vi "niScope EX Configured Acquisition_V3.vi"() -> ()   [LabVIEW 2024]
doc: "Recommended Input Signal: 100 kHz, 4 Vpp, sine wave\n\nDevices Supported: Refer to NI Example Finder\n\nThis example configures all the oscilloscope's vertical, horizontal, and triggering properties before every acquisition. It allows you to experiment with numerous configurations, including acquisition types and triggering modes, since it supports nearly the entire functionality of NI-SCOPE. However, it is may be more instructive to consult other examples about specific topics such as FlexRes, Random Interleaved Sampling, and Multi-Record to learn more about these features.\n\nMany parameters are included an the front panel of this example. Notice that the \"min sample rate\" is next to the \"actual sample rate,\" and similarly the \"min record length\" is near the \"actual record length.\" The \"min\" values are specified with the Configure Horizontal Timing VI. NI-SCOPE maintains a constant time per record for each acquisition. So when you specify a min sample rate and a min record length, this determines the amount of time the acquisition should take:\n\n time per record = min record length / min sampling rate. \n\nHowever, oscilloscopes support only a certain number of defined sampling rates, so if the value chosen is not a valid rate, it is rounded to the next higher rate, called the actual sample rate. The actual record length is then calculated in order to maintain the time per record. Both of these values are returned in this example so you can investigate the effects of parameter rounding with your oscilloscope. For more information about parameter coercions, see the NI High Speed Digitizers Help.\n\nThe enforce realtime property allows this example to use Random Interleaved Sampling. See the Random Interleaved Sampling example for more details.\n\nKeep in mind that not all digitizers/oscilloscopes support all the features in this example. The NI High Speed Digitizers Help includes a table of supported features for each device."
uses:
  <instrlib>/niScope/Controls/niScope vertical coupling.ctl
  <instrlib>/niScope/Utility/niScope Get Channel Name From String.vi
  <instrlib>/niScope/Configure/Trigger/niScope Configure Trigger Immediate.vi
  <instrlib>/niScope/Configure/Trigger/niScope Configure Trigger Edge.vi
  <instrlib>/niScope/Configure/Trigger/niScope Configure Trigger Digital.vi
  <instrlib>/niScope/Configure/Trigger/niScope Configure Trigger Window.vi
  <instrlib>/niScope/Configure/Trigger/niScope Configure Trigger Hysteresis.vi
  <instrlib>/niScope/Acquire/Fetch/niScope Multi Fetch WDT.vi
panel:
  out "Waveform Graph 2":waveform(dbl)(graph)
  out "Waveform Graph":waveform(dbl)(graph)
  in  "Trigger Type":T1(tab)
  in  "Trigger Source":string(combo)="0"
  in  "Trigger Level":dbl format="%.2f"
  in  "Trigger Slope":i32(ring) items=["Positive", "Negative"]
  in  "Coupling":u16(ring)=1 caption="Trigger Coupling" items=["AC"=0, "DC"=1, "HF Reject"=3, "LF Reject"=4, "AC Plus HF Reject"=1001]
  in  "Trigger Slope":i32(ring) items=["Positive", "Negative"]
  in  "Trigger Source":string(combo)="VAL_PFI_1"
  in  "Coupling":u16(ring)=1 caption="Trigger Coupling" items=["AC"=0, "DC"=1, "HF Reject"=3, "LF Reject"=4, "AC Plus HF Reject"=1001]
  in  "High Level":dbl=0.1 caption="Window High Level" format="%.2f"
  in  "Low Level":dbl=-0.1 caption="Window Low Level" format="%.2f"
  in  "Window Mode":i32(ring) items=["Entering", "Leaving"]
  in  "Trigger Source":string(combo)="0"
  in  "Hysteresis":dbl=0.05 format="%.2f"
  in  "Trigger Source":string(combo)="0"
  in  "Trigger Level":dbl format="%.2f"
  in  "Coupling":u16(ring)=1 caption="Trigger Coupling" items=["AC"=0, "DC"=1, "HF Reject"=3, "LF Reject"=4, "AC Plus HF Reject"=1001]
  in  "Trigger Slope":i32(ring) items=["Positive", "Negative"]
  out "Auto Triggered":bool
  in  "Trigger Modifier":i32(ring)=2 items=["None"=1, "Auto Trigger"=2]
  in  "Stop":bool
  in  "Reference Position":dbl=50.0 caption="Ref Position" format="%.1f"
  in  "Trigger Delay":dbl caption="Trigger Delay (s)" format="%#.4p"
  in  "Maximum Input Frequency":dbl caption="Max. Input Frequency (Hz)" format="%.2f"
  in  "Input Impedance":u32(ring) items=["1 mega ohm"=0, "50 ohms"=2]
  in  "Vertical Offset":dbl caption="Vertical Offset (V)" format="%.2p"
  out "Actual Sample Rate":dbl=10000000.0 format="%#.2p"
  out "Actual Record Length":i32=1000
  in  "Min Record Length":i32=1000 caption="Min. Record Length"
  in  "Min Sample Rate":dbl=10000000.0 caption="Min. Sample Rate" step=1000000.0 format="%#.2p"
  in  "Vertical Range":dbl=5.0 caption="Vertical Range (V)" format="%.2f"
  in  "Enforce Realtime":bool=TRUE
  in  "Channel Name":string="0" caption="Channel(s)"
  in  "Resource Name":refnum<k15>="Dev1" caption="Resource Name(s)"
  # "Vertical"
  # "Channel"
  # "Trigger"
  # "Common Trigger Settings"
  # "Horizontal"
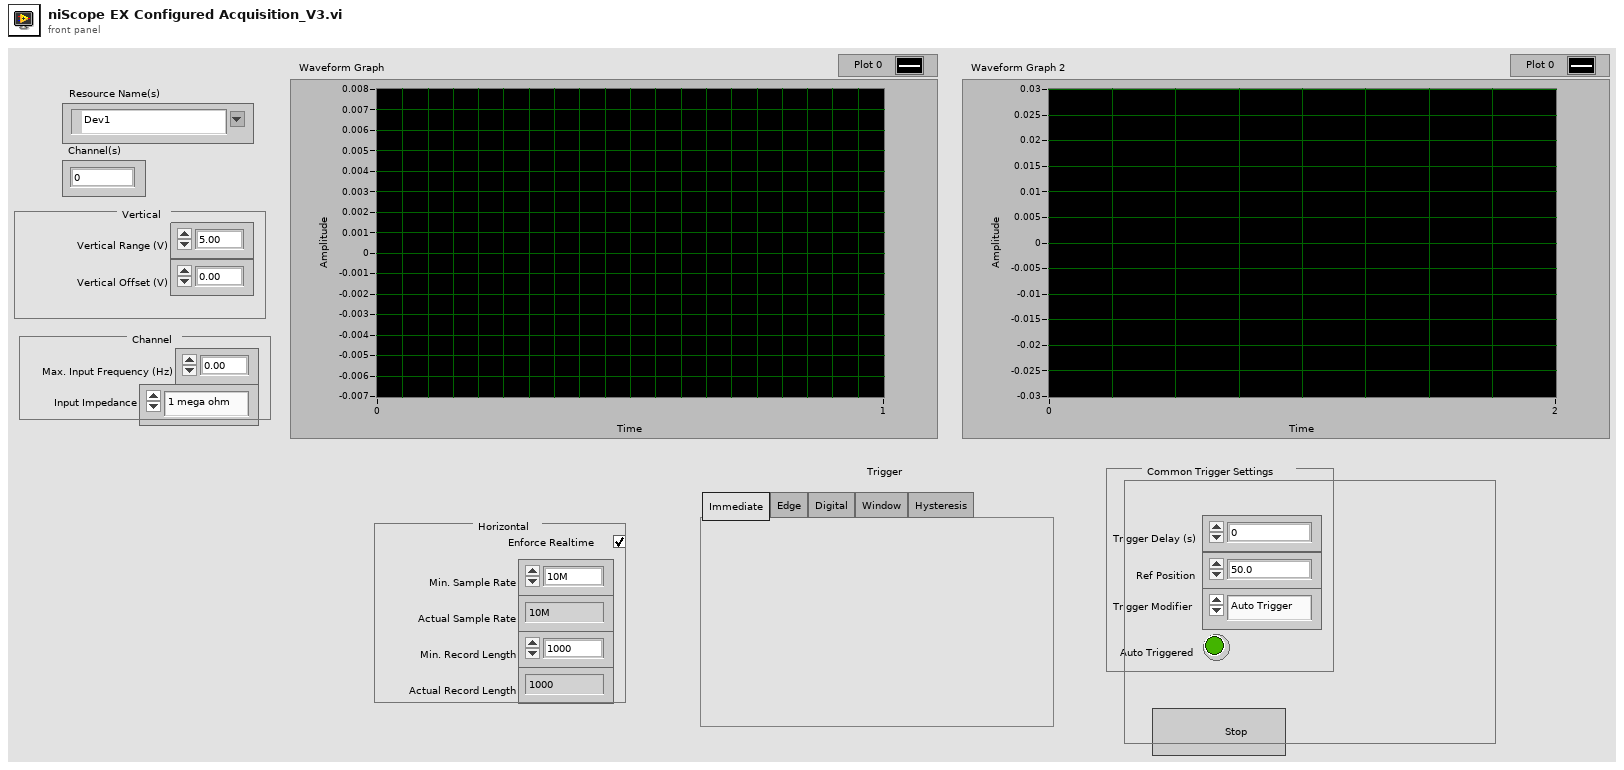
[diagram p1: front panel]
types:
  T1 = enum32{"Immediate", "Edge", "Digital", "Window", "Hysteresis"}
  T2 = enum16{"open", "open or create", "create or replace", "create", "open (read-only)"}
  T3 = typedef "niScope vertical coupling.ctl" = i32
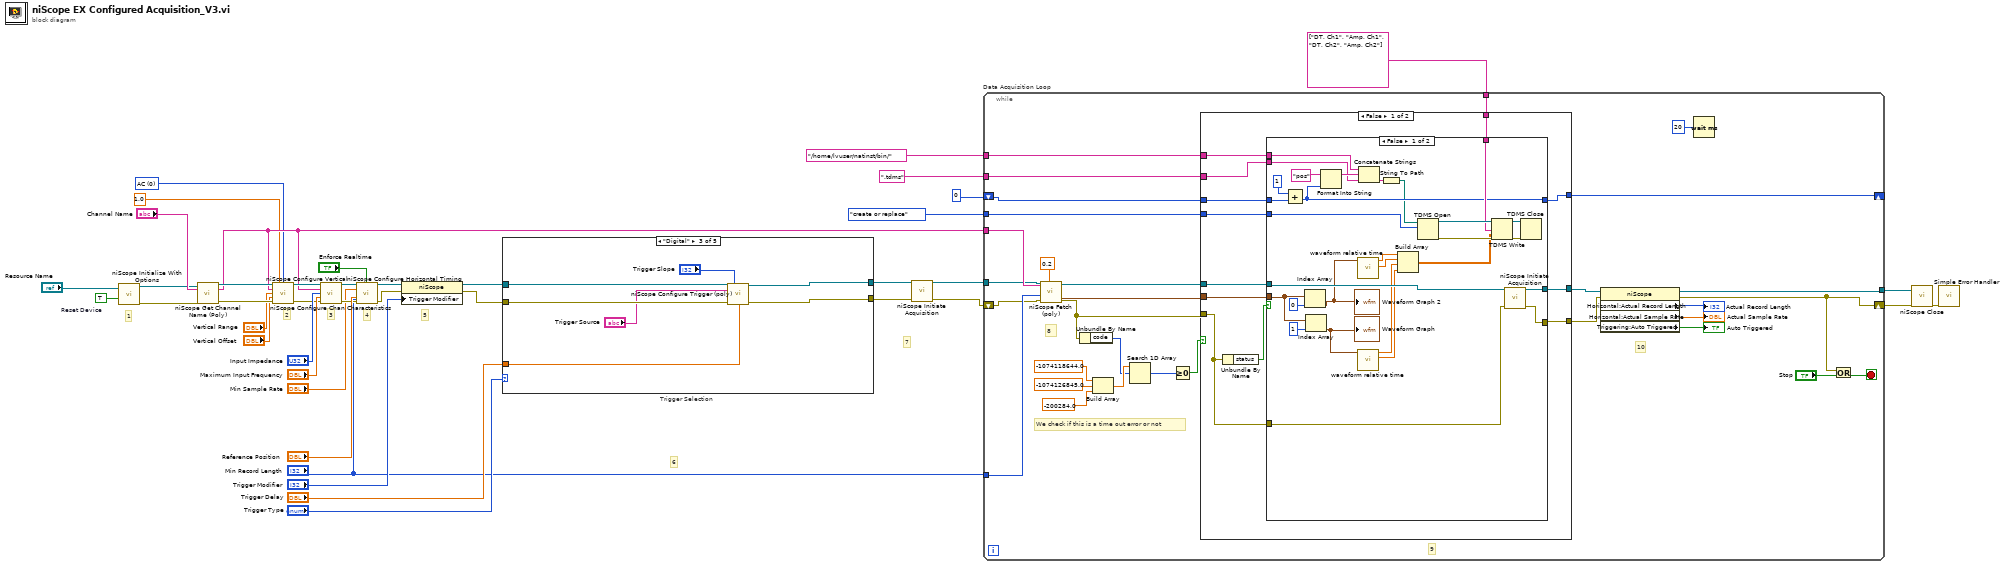
[diagram p0: block diagram]
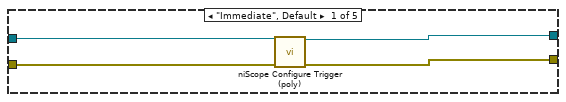
[diagram p2: hidden frame]
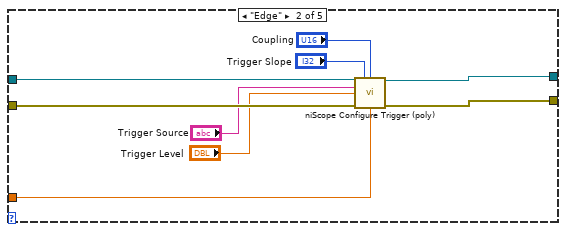
[diagram p3: hidden frame]
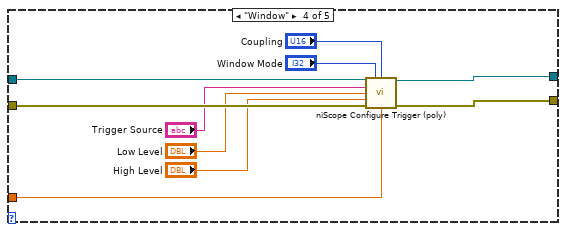
[diagram p4: hidden frame]
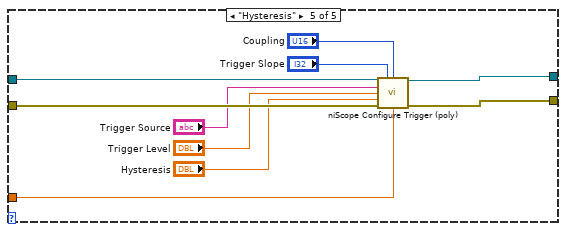
[diagram p5: hidden frame]
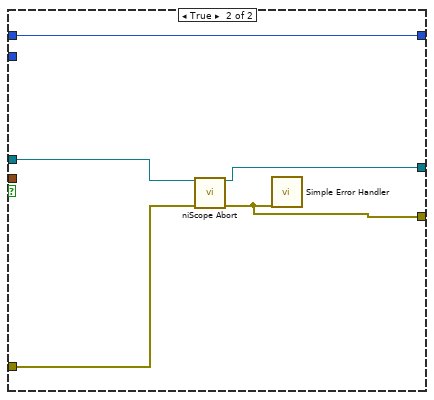
[diagram p6: hidden frame]
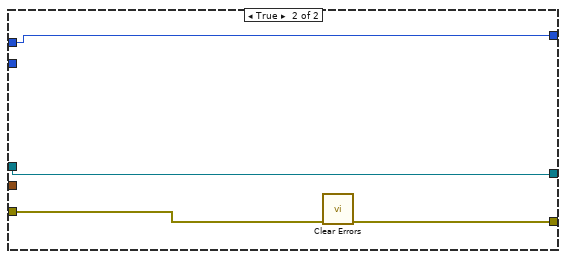
[diagram p7: hidden frame]
diagram:
  w7 = T3 0 items=["AC", "DC", "Ground"] ("vertical coupling")
  w41 = TRUE  # Reset Device
  # "5"
  # "2"
  # "3"
  # "4"
  # "6"
  # "7"
  # "1"
  n1 = call <instrlib>:"niScope Initialize With Options.vi"("resource name"="Resource Name", "reset device"=w41) -> ("instrument handle"=w13:refnum<k15>, "error out"=w12:errorcluster)  [unwired: 12 in]
  n2 = call-poly <instrlib>:"niScope Get Channel Name (Poly).vi"("instrument handle"=w13, "index"="Channel Name", "error in"=w12) -> ("instrument handle out"=w34:refnum<k15>, "channel name"=w11:string, "error out"=w35:errorcluster)  [unwired: 10 in]
  n3 = call <instrlib>:"niScope Configure Vertical.vi"("instrument handle"=w34, "probe attenuation"=1.0, "vertical coupling"=w7, "channels"=w11, "vertical range"="Vertical Range", "vertical offset"="Vertical Offset", "error in"=w35) -> ("instrument handle out"=w16:refnum<k15>, "error out"=w17:errorcluster)  [unwired: 7 in]
  n4 = call <instrlib>:"niScope Configure Chan Characteristics.vi"("instrument handle"=w16, "channels"=w11, "input impedance"="Input Impedance", "maximum input frequency"="Maximum Input Frequency", "error in"=w17) -> ("instrument handle out"=w19:refnum<k15>, "error out"=w18:errorcluster)  [unwired: 9 in]
  n5 = call <instrlib>:"niScope Configure Horizontal Timing.vi"("instrument handle"=w19, "enforce realtime"="Enforce Realtime", "min sample rate"="Min Sample Rate", "reference position"="Reference Position", "error in"=w18, "min record length"="Min Record Length") -> ("instrument handle out"=w27:refnum<k15>, "error out"=w28:errorcluster)  [unwired: 8 in]
  n6 = property on="Property Node" class="niScope"(reference=w27, error in=w28, "Trigger Modifier"="Trigger Modifier") -> (reference out=w30:refnum<k15>, error out=w29:errorcluster)
  n7 = case "Trigger Selection" shown="\"Digital\"" "Trigger Type" {
    tunnel: w29 -> [w45 w54 w61 w71 w81]
    tunnel: [w42 w50 w57 w67 w77] -> w26
    tunnel: w30 -> [w44 w53 w60 w70 w80]
    tunnel: [w43 w51 w58 w68 w79] -> w25
    tunnel: "Trigger Delay" -> [_ w52 w59 w69 w78]
    frame "Immediate", Default {
      n8 = call-poly <instrlib>:"niScope Configure Trigger (poly).vi"("instrument handle"=w44, "error in"=w45) -> ("instrument handle out"=w43:refnum<k15>, "error out"=w42:errorcluster)  [unwired: 12 in]
    }
    frame "Edge" {
      n9 = call-poly <instrlib>:"niScope Configure Trigger (poly).vi"("instrument handle"=w53, "trigger slope"="Trigger Slope", "trigger coupling"="Coupling", "trigger source"="Trigger Source", "trigger level"="Trigger Level", "error in"=w54, "trigger delay"=w52) -> ("instrument handle out"=w51:refnum<k15>, "error out"=w50:errorcluster)  [unwired: 7 in]
    }
    frame "Digital" {
      n10 = call-poly <instrlib>:"niScope Configure Trigger (poly).vi"("instrument handle"=w60, "trigger slope"="Trigger Slope", "trigger source"="Trigger Source", "error in"=w61, "trigger delay"=w59) -> ("instrument handle out"=w58:refnum<k15>, "error out"=w57:errorcluster)  [unwired: 9 in]
    }
    frame "Window" {
      n11 = call-poly <instrlib>:"niScope Configure Trigger (poly).vi"("instrument handle"=w70, "trigger window mode"="Window Mode", "trigger coupling"="Coupling", "trigger source"="Trigger Source", "low level"="Low Level", "high level"="High Level", "error in"=w71, "trigger delay"=w69) -> ("instrument handle out"=w68:refnum<k15>, "error out"=w67:errorcluster)  [unwired: 6 in]
    }
    frame "Hysteresis" {
      n12 = call-poly <instrlib>:"niScope Configure Trigger (poly).vi"("instrument handle"=w80, "trigger slope"="Trigger Slope", "trigger coupling"="Coupling", "trigger source"="Trigger Source", "trigger level"="Trigger Level", "hysteresis"="Hysteresis", "error in"=w81, "trigger delay"=w78) -> ("instrument handle out"=w79:refnum<k15>, "error out"=w77:errorcluster)  [unwired: 6 in]
    }
  }
  n13 = call <instrlib>:"niScope Initiate Acquisition.vi"("instrument handle"=w25, "error in"=w26) -> ("instrument handle out"=w10:refnum<k15>, "error out"=w8:errorcluster)  [unwired: 12 in]
  n14 = while "Data Acquisition Loop" {
    tunnel: [w112] -> w39
    shift-right: [w106] -> w38
    shift-left: w8 -> [w88]
    tunnel: w11 -> [w91]
    tunnel: w10 -> [w90]
    tunnel: "Min Record Length" -> [w89]
    tunnel: string[] ["DT, Ch1", "Amp, Ch1", "DT, Ch2", "Amp, Ch2"] ("channel name(s) in (Untitled)") -> [w87]
    tunnel: "/home/lvuser/natinst/bin/" ("string") -> [w86]
    tunnel: ".tdms" ("string") -> [w85]
    tunnel: T2."create or replace" ("operation (0:open)") -> [w84]
    shift-right: [w82] -> _
    shift-left: 0 -> [w83]
    stop <- w107 stop-if-true
    # "9"
    # "We check if this is a time out error or not"
    # "8"
    # "10"
    n15 = call-poly <instrlib>:"niScope Fetch (poly).vi"("timeout"=0.2, "error in"=w88, "numSamples"=w89, "channels"=w91, "instrument handle"=w90) -> ("error out"=w98:errorcluster, "wfm"=w94:waveform(dbl)[], "instrument handle out"=w96:refnum<k15>)  [unwired: 3 in, 1 out]
    n16 = Unbundle By Name(w98) -> ("code"=w92:i32)
    n17 = Build Array(-1074118644.0 ("element"), -1074126845.0 ("element"), -200284.0 ("element")) -> (w101:dbl[])
    n18 = Search 1D Array(1D array=w101, element=w92) -> (index of element=w100:i32)  [unwired: 1 in]
    n19 = Greater Or Equal To 0?(x=w100) -> (x >= 0?=w99:bool)
    n20 = case shown="False" w99 {
      tunnel: w98 -> [w120 w162]
      tunnel: [w123 w161] -> w97
      tunnel: w96 -> [w122 w161]
      tunnel: [w121 w160] -> w95
      tunnel: w94 -> [w119 _]
      tunnel: w87 -> [w118 _]
      tunnel: w86 -> [w115 _]
      tunnel: w85 -> [w114 _]
      tunnel: [w117 w159] -> w82
      tunnel: w84 -> [w116 _]
      tunnel: w83 -> [w113 w159]
      frame False {
        n21 = Unbundle By Name(w120) -> ("status"=w124:bool)
        n22 = case shown="False" w124 {
          tunnel: [w152 w157] -> w123
          tunnel: w122 -> [w153 w158]
          tunnel: [w150 w155] -> w121
          tunnel: w120 -> [w151 w156]
          tunnel: w119 -> [w141 _]
          tunnel: w118 -> [w148 _]
          tunnel: [w131 w154] -> w117
          tunnel: w116 -> [w129 _]
          tunnel: w115 -> [w128 _]
          tunnel: w114 -> [w127 _]
          tunnel: w113 -> [w126 w154]
          frame False {
            n23 = Add(x=1, y=w126) -> (x+y=w131:i32)
            n24 = Index Array(array=w141, index=0) -> (element=w136:waveform(dbl))
            "Waveform Graph 2" <- w136
            n25 = Index Array(array=w141, index=1) -> (element=w139:waveform(dbl))
            "Waveform Graph" <- w139
            n26 = Format Into String(initial string="pos", w131) -> (resulting string=w134:string)  [unwired: 2 in, 1 out]
            n27 = call "waveform relative time.vi"("signal in"=w136) -> ("Y"=w135:dbl[], "Relative Time"=w146:dbl[])  [unwired: 7 in, 2 out]
            n28 = call "waveform relative time.vi"("signal in"=w139) -> ("Y"=w137:dbl[], "Relative Time"=w138:dbl[])  [unwired: 7 in, 2 out]
            n29 = Concatenate Strings(w128, w134, w127) -> (w133:string)
            n30 = String To Path(string=w133) -> (path=w130:path)
            n31 = Build Array(w146, w135, w138, w137) -> (w145:dbl[][])
            n32 = TDMS Open(10:w129, 11:w130) -> (0:w147:errorcluster, 3:w149:refnum<k34>)  [unwired: 5 in]
            n33 = TDMS Write(0:w149, 7:w148, 9:w145, 11:w147) -> (4:w144:refnum<k34>, 15:w143:errorcluster)  [unwired: 2 in, 2 out]
            n34 = call <instrlib>:"niScope Initiate Acquisition.vi"("instrument handle"=w153, "error in"=w151) -> ("instrument handle out"=w152:refnum<k15>, "error out"=w150:errorcluster)  [unwired: 12 in]
            n35 = TDMS Close(8:w143, 11:w144) -> ()  [unwired: 2 out]
          }
          frame True {
            n36 = call <instrlib>:"niScope Abort.vi"("instrument handle"=w158, "error in"=w156) -> ("instrument handle out"=w157:refnum<k15>, "error out"=w155:errorcluster)  [unwired: 12 in]
            n37 = call <vilib>:"Simple Error Handler.vi"("error in (no error)"=w155) -> ()  [unwired: 4 in, 5 out]
          }
        }
      }
      frame True {
        n38 = call <vilib>:"Clear Errors.vi"("error in (no error)"=w162) -> ("error out"=w160:errorcluster)  [unwired: 5 in, 1 out]
      }
    }
    n39 = property class="niScope"(reference=w97, error in=w95) -> (reference out=w112:refnum<k15>, error out=w106:errorcluster, "Horizontal:Actual Record Length"=→"Actual Record Length":i32, "Horizontal:Actual Sample Rate"=→"Actual Sample Rate":dbl, "Triggering:Auto Triggered"=→"Auto Triggered":bool)
    n40 = Wait (ms)(milliseconds to wait=u32 20) -> ()  [unwired: 1 out]
    n41 = Or(x=w106, y="Stop") -> (x .or. y?=w107:bool)
  }
  n42 = call <instrlib>:"niScope Close.vi"("instrument handle"=w39, "error in"=w38) -> ("error out"=w40:errorcluster)  [unwired: 13 in]
  n43 = call <vilib>:"Simple Error Handler.vi"("error in (no error)"=w40) -> ()  [unwired: 4 in, 5 out]
